vi "execCL.vi"(8 "error in (no error)":errorcluster, 10 "command line":string) -> (0 "error out":errorcluster, 1 "return code":i32, 2 "standard output":string, 4 "standard error":string)   [LabVIEW 2016]
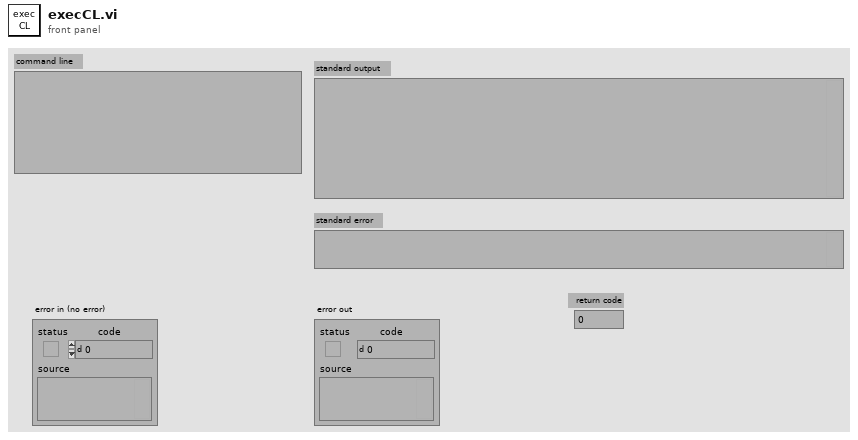
[diagram p1: front panel]
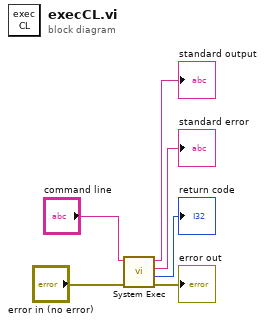
[diagram p0: block diagram]
diagram:
  n1 = call <vilib>:"System Exec.vi"("error in (no error)"="error in (no error)", "command line"="command line") -> ("error out"=→"error out":errorcluster, "return code"=→"return code":i32, "standard error"=→"standard error":string, "standard output"=→"standard output":string)  [unwired: 6 in]
